vi "Get Loop Time (ms).vi"() -> (0 "Loop Time":u32)   [LabVIEW 2016]
panel:
  # "This VI returns the time difference between sucessive calls.\nUsing a feedback node without a loop was made possible in LabVIEW 8.5."
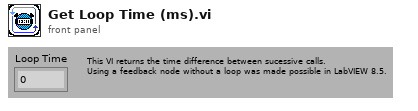
[diagram p1: front panel]
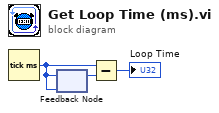
[diagram p0: block diagram]
diagram:
  n1 = Tick Count (ms)() -> (millisecond timer value=w2:u32)
  n2 = feedback-in #1(w2) -> ()
  n3 = feedback #1(w2) -> (w1:u32)
  n4 = Subtract(x=w2, y=w1) -> (x-y=→"Loop Time":u32)
